vi "MGI RWA List Sections.vi"(8 "error in":errorcluster, 11 "Path (dialog)":path=path "C:/Users/Brandon/Desktop/deleteme.ini") -> (0 "error out":errorcluster, 2 "Section[]":string[](array[string]))   [LabVIEW 2020]
doc: "Returns all the section names in a Read/Write Anything file.\n\nAuthor: Brandon D. Steele\n\nFreeware from Moore Good Ideas, www.mooregoodideas.com. Do not remove this line."
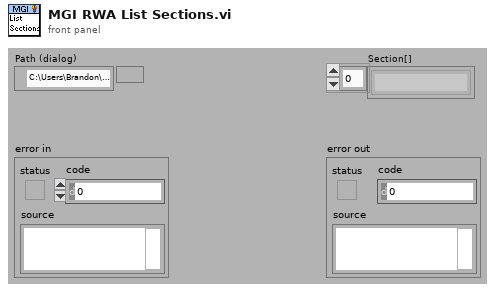
[diagram p1: front panel]
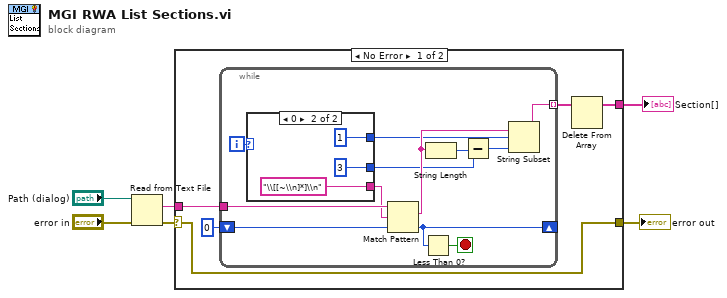
[diagram p0: block diagram]
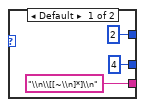
[diagram p2: hidden frame]
diagram:
  n1 = Read from Text File(file (use dialog)="Path (dialog)", error in="error in") -> (text=w2:string, error out=w1:errorcluster)  [unwired: 4 out]
  n2 = case shown="No Error" w1 {
    selector: w1 -> [w7 w30]
    tunnel: w2 -> [w11 _]
    tunnel: [w8 _] -> w5
    tunnel: [w7 w30] -> w4
    frame No Error {
      n3 = while {
        tunnel: w11 -> [w23]
        shift-right: [w21] -> _
        shift-left: 0 ("offset past match") -> [w22]
        tunnel: [w12] -> w9 mode=indexing
        i -> [w16]
        stop <- w20 stop-if-true
        n4 = case shown="0" w16 {
          tunnel: ["\\n\\[[~\\n]*]\\n" ("regular expression") "\\[[~\\n]*]\\n" ("regular expression")] -> w15
          tunnel: [2 ("offset (0)") 1 ("offset (0)")] -> w13
          tunnel: [4 ("y") 3 ("y")] -> w14
          frame Default {
          }
          frame 0 {
          }
        }
        n5 = Match Pattern(string=w23, regular expression=w15, offset (0)=w22) -> (match substring=w18:string, offset past match=w21:i32)  [unwired: 2 out]
        n6 = Less Than 0?(x=w21) -> (x < 0?=w20:bool)
        n7 = String Length(string=w18) -> (length=w19:i32)
        n8 = Subtract(x=w19, y=w14) -> (x-y=w17:i32)
        n9 = String Subset(string=w18, offset (0)=w13, length (rest)=w17) -> (substring=w12:string)
      }
      n10 = Delete From Array(array=w9) -> (array with subset deleted=w8:string[])  [unwired: 2 in, 1 out]
    }
    frame Error {
    }
  }
  "Section[]" <- w5
  "error out" <- w4
